vi "Pre Launch Init.vi"(11 "FirstActor in":refnum<class "FirstActor.lvclass">) -> (0 "error out":errorcluster, 3 "FirstActor out":refnum<class "FirstActor.lvclass">)   [LabVIEW 2020, in "FirstActor.lvlib" / "FirstActor.lvclass"]
doc: "(<B>Filename</B>: Actor Framework.lvlib:Actor.lvclass:Pre Launch Init.vi)\n\nDefines behavior that occurs after the Launch Nested Actor method is invoked but before the actor's Actor Core method begins running.\n\nBy default, this method does nothing. A descendant class may override it to define behavior."
uses:
  FirstActor.lvclass
  C:/Program Files (x86)/National Instruments/LabVIEW 2020/vi.lib/ActorFramework/Actor/Actor.lvclass
  <vilib>/ActorFramework/Actor/Actor.lvclass/Actor.ctl
  <vilib>/ActorFramework/Message Enqueuer/Message Enqueuer.lvclass/Message Enqueuer.ctl
  <vilib>/ActorFramework/Message Enqueuer/Enqueue.vi
  <vilib>/ActorFramework/Message Enqueuer/Init from Existing Queue.vi
  FirstActor Messages/Inicializar Fecha Msg/Inicializar Fecha Msg.lvclass
  C:/Program Files (x86)/National Instruments/LabVIEW 2020/vi.lib/ActorFramework/Message/Message.lvclass
  <vilib>/ActorFramework/Message Priority Queue/Priority Enqueue.vi
  <vilib>/ActorFramework/Actor/Actor.lvclass
  <vilib>/ActorFramework/Message Enqueuer/Message Enqueuer.lvclass
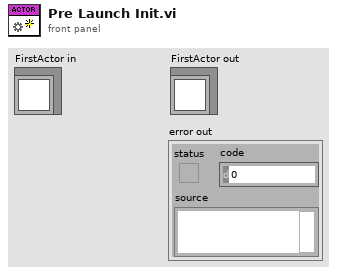
[diagram p1: front panel]
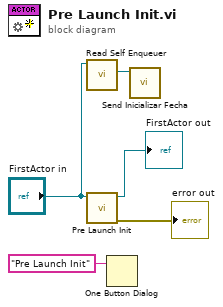
[diagram p0: block diagram]
diagram:
  n1 = call <vilib>:"Read Self Enqueuer.vi"("Actor"="FirstActor in") -> ("Self Enqueuer"=w1:refnum<class "Message Enqueuer.lvclass">)  [unwired: 10 in]
  n2 = call-parent "Pre Launch Init.vi"("Actor in"="FirstActor in") -> ("error out"=→"error out":errorcluster, "Actor out"=→"FirstActor out":refnum<class "FirstActor.lvclass">)  [unwired: 9 in]
  n3 = One Button Dialog(message="Pre Launch Init") -> ()  [unwired: 1 in, 1 out]
  n4 = call "Send Inicializar Fecha.vi"("Message Enqueuer"=w1) -> ()  [unwired: 9 in, 2 out]
